vi "Get_ADC_conversion_factors.vi"(1 "Strings":string[](array[string])) -> (0 "Conversion factors":dbl[](array[numeric]))   [LabVIEW 2013]
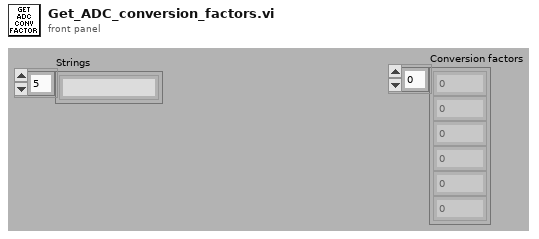
[diagram p1: front panel]
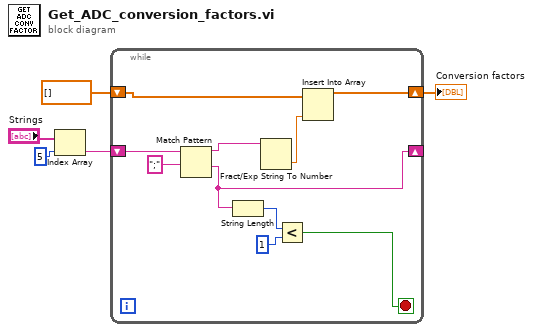
[diagram p0: block diagram]
diagram:
  n1 = Index Array(array="Strings", index=5) -> (element=w3:string)
  n2 = while {
    shift-right: [w8] -> w1
    shift-left: dbl[] [] -> [w9]
    shift-right: [w6] -> _
    shift-left: w3 -> [w15]
    stop <- w10 stop-if-true
    n3 = Match Pattern(string=w15, regular expression=";") -> (before substring=w13:string, after substring=w6:string)  [unwired: 1 in, 2 out]
    n4 = String Length(string=w6) -> (length=w12:i32)
    n5 = Fract/Exp String To Number(string=w13) -> (number=w7:dbl)  [unwired: 3 in, 1 out]
    n6 = Less?(x=w12, y=1) -> (x < y?=w10:bool)
    n7 = Insert Into Array(array=w9, new element=w7) -> (w8:dbl[])  [unwired: 1 in]
  }
  "Conversion factors" <- w1
